vi "GenAngle.vi"(8 "Min Stroke":i32, 9 "Max Stroke":i32, 11 "Force In":dbl[](array[numeric])) -> (0 "Last Angle":dbl, 3 "Angle Out":dbl[](array[numeric]))   [LabVIEW 2017]
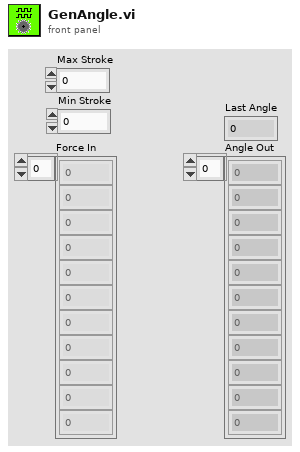
[diagram p1: front panel]
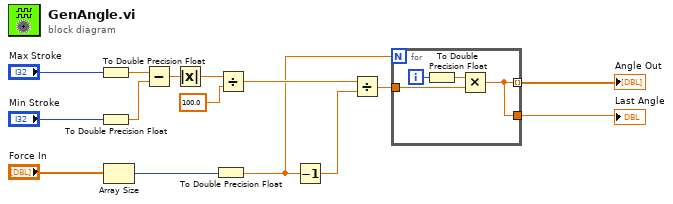
[diagram p0: block diagram]
diagram:
  n1 = To Double Precision Float(number="Max Stroke") -> (double precision float=w15:dbl)
  n2 = To Double Precision Float(number="Min Stroke") -> (double precision float=w14:dbl)
  n3 = Array Size(array="Force In") -> (size(s)=w4:i32)
  n4 = Subtract(x=w15, y=w14) -> (x-y=w11:dbl)
  n5 = Absolute Value(x=w11) -> (abs(x)=w13:dbl)
  n6 = To Double Precision Float(number=w4) -> (double precision float=w2:dbl)
  n7 = Divide(x=w13, y=100.0) -> (x/y=w10:dbl)
  n8 = Decrement(x=w2) -> (x-1=w5:dbl)
  n9 = Divide(x=w10, y=w5) -> (x/y=w6:dbl)
  n10 = for {
    N: w2 -> [_]
    tunnel: w6 -> [w19]
    tunnel: [w16] -> w3 mode=indexing
    tunnel: [w16] -> w1
    i -> [w17]
    n11 = To Double Precision Float(number=w17) -> (double precision float=w18:dbl)
    n12 = Multiply(x=w18, y=w19) -> (x*y=w16:dbl)
  }
  "Angle Out" <- w3
  "Last Angle" <- w1
